vi "Actor Core.vi"(8 "error in":errorcluster, 11 "Test Executive Builder ViewManager In":refnum<class "Test Executive Builder ViewManager.lvclass">) -> (0 "error out":errorcluster, 3 "Actor out":refnum<class "Actor.lvclass">)   [LabVIEW 2017, in "Test Executive Builder ViewManager.lvclass"]
doc: "(<B>Filename</B>: Actor Framework.lvlib:Actor.lvclass:Actor Core.vi)\n\nReceives messages to the actor, reacts to them, and initiates any error handling that may shut the actor down.\n\nDescendant classes may override this VI to append parallel tasks for the actor to complete while it handles messages. Overrides use the Call Parent Method node.\n\n<License>\nCopyright © 2017 Composed Systems, LLC | All rights reserved\nwww.composed.io\n\nAuthor: Ethan Stern <ethan.stern@composed.io>\n\nThis software is provided \"AS IS\" WITHOUT WARRANTIES, either express or implied, AND IS FOR EDUCATIONAL PURPOSES ONLY.\n</License>"
uses:
  Test Executive Builder ViewManager.lvclass
  <vilib>/ActorFramework/Actor/Actor.lvclass
  Test Executive Builder ViewManager.lvclass/Test Executive Builder ViewManager.ctl
  <vilib>/gpm_packages/@cs/mva-viewable/Source/IViewManager/IViewManager/IViewManager.lvclass
  <vilib>/gpm_packages/@cs/mva-viewable/Source/IViewable/ProtectedSubpanel/ProtectedSubpanel.lvclass
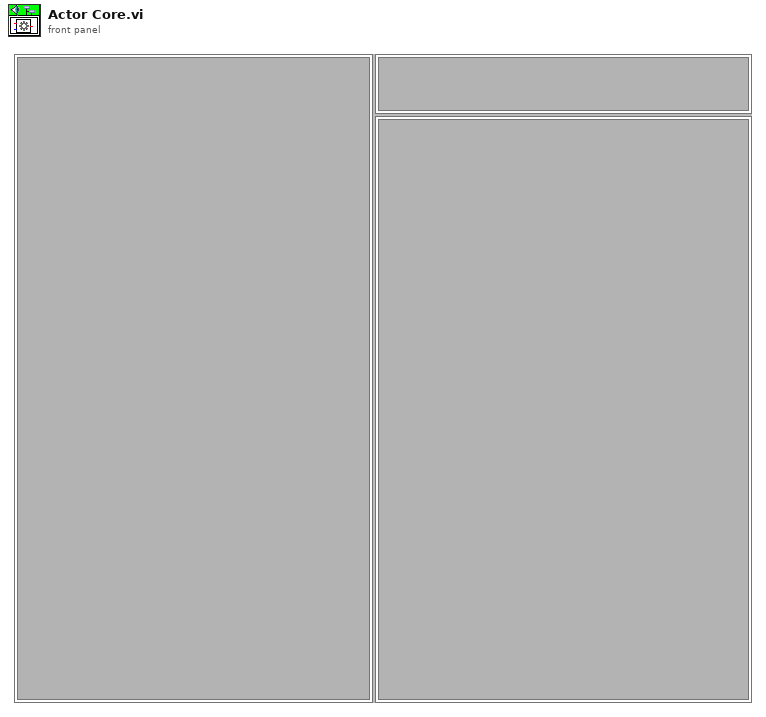
[diagram p1: front panel]
types:
  T1 = typedef "IViewable.lvlib/ProtectedSubpanel.lvclass/Protected Subpanel Reference.ctl" = refnum<data-value>
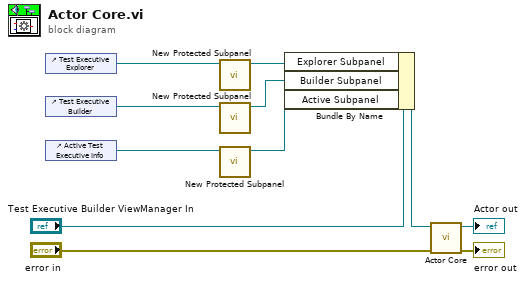
[diagram p0: block diagram]
diagram:
  n1 = control-ref of="Test Executive Explorer"() -> (w7:refnum<vi>)
  n2 = control-ref of="Test Executive Builder"() -> (w8:refnum<vi>)
  n3 = control-ref of="Active Test Executive Info"() -> (w2:refnum<vi>)
  n4 = call <vilib>:"New Protected Subpanel.vi"("SubPnl Refnum"=w7) -> ("Protected Subpanel"=w4:T1)  [unwired: 9 in, 1 out]
  n5 = call <vilib>:"New Protected Subpanel.vi"("SubPnl Refnum"=w8) -> ("Protected Subpanel"=w3:T1)  [unwired: 9 in, 1 out]
  n6 = call <vilib>:"New Protected Subpanel.vi"("SubPnl Refnum"=w2) -> ("Protected Subpanel"=w1:T1)  [unwired: 9 in, 1 out]
  n7 = Bundle By Name(cluster="Test Executive Builder ViewManager In", "Explorer Subpanel"=w4, "Builder Subpanel"=w3, "Active Subpanel"=w1) -> (w5:refnum<class "Test Executive Builder ViewManager.lvclass">)
  n8 = call-parent "Actor Core.vi"("error in"="error in", "IViewable In"=w5) -> ("error out"=→"error out":errorcluster, "Actor out"=→"Actor out":refnum<class "Actor.lvclass">)  [unwired: 8 in]
